vi "Configure Trigger.vi"(8 "error in (no error)":errorcluster, 9 "Trigger Time (1 s)":dbl=1.0 min=1.0 max=999.99 step=0.01 format="%.2g", 10 "Trigger Source (0:Bus)":u16(ring) items=["Bus", "External", "Hold", "Manual", "Timed"], 11 "VISA resource name":refnum<visa-resource-name>) -> (0 "error out":errorcluster, 3 "VISA resource name out":refnum<visa-resource-name>)   [LabVIEW 2018, in "BK Precision 8600 Series.lvlib"]
doc: "Configures the trigger settings of the instrument. This VI should be used before sending any trigger to the instrument from any source."
uses:
  <instrlib>/BK Precision 8600 Series/BK Precision 8600 Series.lvlib
panel:
  # "s"
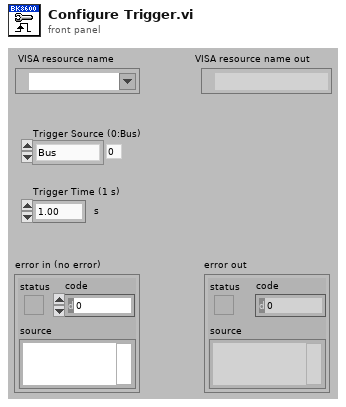
[diagram p1: front panel]
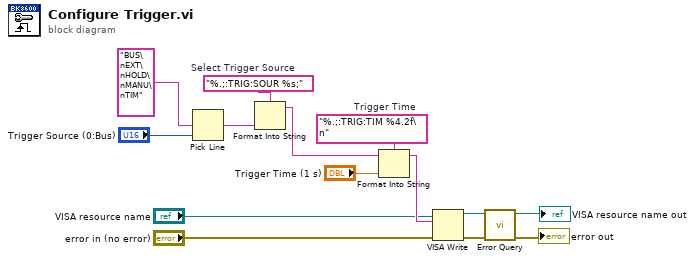
[diagram p0: block diagram]
diagram:
  w8 = "%.;:TRIG:SOUR %s;"  # Select Trigger Source
  w10 = "%.;:TRIG:TIM %4.2f\n"  # Trigger Time
  n1 = Pick Line(multi-line string="BUS\nEXT\nHOLD\nMANU\nTIM", line index="Trigger Source (0:Bus)") -> (output string=w6:string)  [unwired: 1 in]
  n2 = Format Into String(format string=w8, w6) -> (resulting string=w4:string)  [unwired: 2 in, 1 out]
  n3 = Format Into String(format string=w10, initial string=w4, "Trigger Time (1 s)") -> (resulting string=w3:string)  [unwired: 1 in, 1 out]
  n4 = VISA Write(VISA resource name="VISA resource name", write buffer=w3, error in (no error)="error in (no error)") -> (VISA resource name out=w13:refnum<visa-resource-name>, error out=w14:errorcluster)  [unwired: 1 out]
  n5 = call <instrlib>:"Error Query.vi"("error in (no error)"=w14, "VISA resource name"=w13) -> ("error out"=→"error out":errorcluster, "VISA resource name out"=→"VISA resource name out":refnum<visa-resource-name>)  [unwired: 6 in, 2 out]
